vi "Boolean_LED.vi"() -> ()   [LabVIEW 2020]
panel:
  out "Output LED":bool
  in  "Input Switch":bool
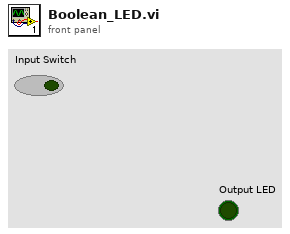
[diagram p1: front panel]
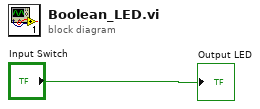
[diagram p0: block diagram]
diagram:
  "Output LED" <- "Input Switch"
